vi "stepper controller -- IMS -- launch progress monitor.vi"(8 "talkback  user event":refnum<user-event>, 11 "talkto user event":refnum<user-event>) -> (2 "reference out":refnum<vi>)   [LabVIEW 2018]
uses:
  stepper monitor message.ctl
  stepper motor state.ctl
  talkto async routine actionn.ctl
panel:
  in  "set step !":dbl(slide)=7372.340425531916 min=0.0 max=16000.0 scale=0.0..16500.0 scale format="%^#6_6g"
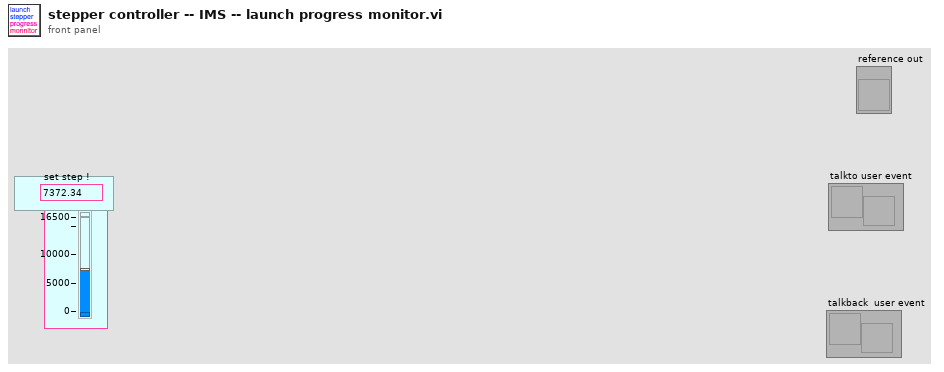
[diagram p1: front panel]
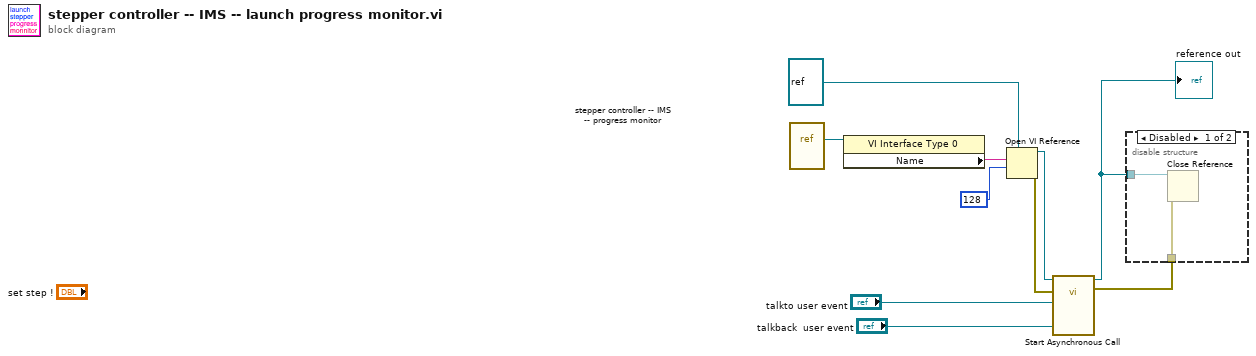
[diagram p0: block diagram]
diagram:
  n1 = vi-ref "stepper controller -- IMS -- progress monitor.vi"() -> (w8:refnum<vi>)
  n2 = property class="VI Interface Type 0"(reference=w8) -> ("Name"=w7:string)  [unwired: 1 in, 2 out]
  n3 = Open VI Reference(type specifier VI Refnum (for type only)=refnum<vi> refnum, vi path=w7, options=128) -> (vi reference=w9:refnum<vi>, error out=w3:errorcluster)  [unwired: 3 in]
  n4 = call-by-ref "Start Asynchronous Call"(reference=w9, error in=w3, "talkback user event"="talkback  user event", "talkto user event"="talkto user event") -> (reference out=w4:refnum<vi>, error out=w5:errorcluster)  [unwired: 10 in]
  "reference out" <- w4
  n5 = disable-structure shown="Disabled" {
    disable-tunnel: w5 -> [w12 _]
    disable-tunnel: w4 -> [w11 _]
    frame Disabled {
      n6 = Close Reference(reference=w11, error in (no error)=w12) -> ()  [unwired: 1 out]
    }
    frame Enabled {
    }
  }
